vi "Counter (Periodic Tasks).vi"(8 "error in":errorcluster) -> ()   [LabVIEW 2011]
doc: "This VI runs in parallel to other tasks. It can contain as many user-defined periodic loops as you need. These can carry out PID or other sorts of timed response."
uses:
  <vilib>/Rock Robotics/WPI/DriverStation/WPI_DriverStationRobotMode.ctl
  Robot Global Data.vi
  <vilib>/addons/control/pid/pid.llb/PID Control Input Filter (DBL).vi
  <vilib>/addons/control/pid/pid.llb/PID (DBL).vi
  <vilib>/addons/control/pid/NI_PID_pid.lvlib
panel:
  out "Allow Fire":dbl(graph)
  out "Current RPM":dbl(graph)
  in  "Graph Enabled":bool
  out "Counter Value":i32
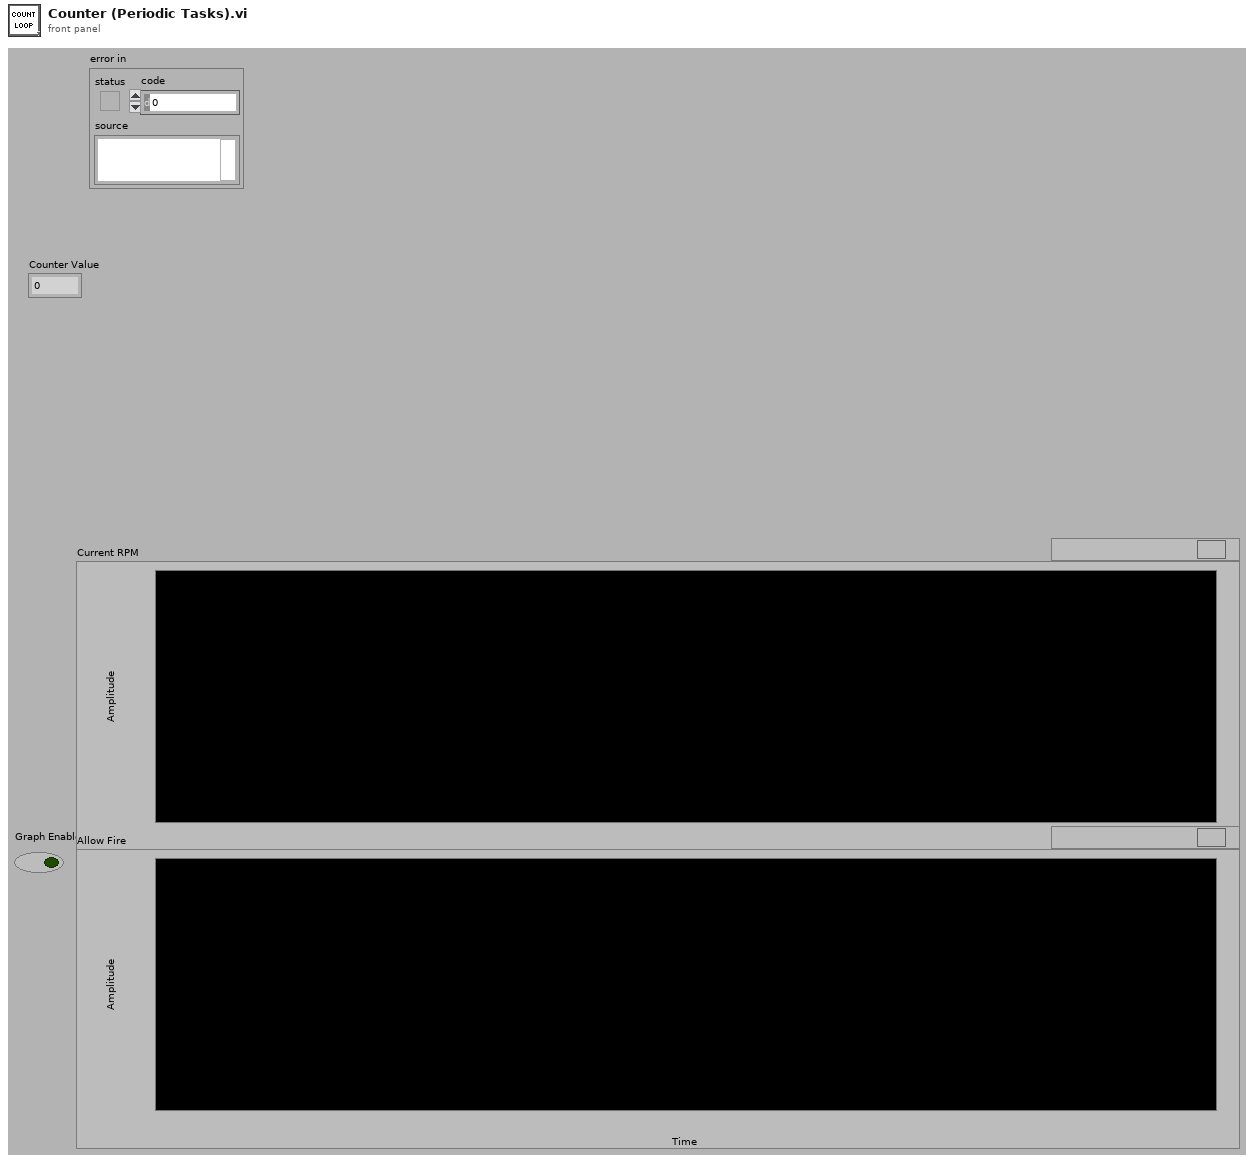
[diagram p1: front panel]
types:
  T1 = typedef "WPI_MotorControlDeviceRef.ctl" = cluster{"DeviceStatus":errorcluster, "Type":enum16{"PWM", "CAN"}, "PWM":cluster{"Digital Module":T2, "PWM Channel":T3, "DeadBand":T4}, "CAN":cluster{"Device Number":u8, "Control Mode":T5, "Semaphore":T6, "Max Vout":dbl}, "Invert":bool, "TransformRef":T7, "InvTransformRef":T7}
  T2 = typedef "FPGA_TypedefDigitalModule.ctl" = enum16{"Digital Module 1", "Digital Module 2"}
  T3 = typedef "FPGA_DIOPWMChannel.ctl" = enum8{"PWM 1", "PWM 2", "PWM 3", "PWM 4", "PWM 5", "PWM 6", "PWM 7", "PWM 8", "PWM 9", "PWM 10", "Invalid"}
  T4 = typedef "WPI_PWMDeadband.ctl" = cluster{"Name":string, "maxPositivePwm":i32, "minPositivePwm":i32, "centerPwm":i32, "maxNegativePwm":i32, "minNegativePwm":i32, "angularRange":u16}
  T5 = typedef "WPI_CANJaguar_ControlMode.ctl" = enum8{"Percent VBus", "Current", "Speed", "Position", "Voltage"}
  T6 = typedef "Semaphore RefNum" = refnum<k1>
  T7 = typedef "WPI_PWMTransform_ConPane.ctl" = refnum<vi>
  T8 = typedef "WPI_CounterDevRef.ctl" = cluster{"DevStatus":errorcluster, "CntIndex":T9}
  T9 = typedef "FPGA_CounterCtrSystemIndex.ctl" = enum8{"Ctr 0", "Ctr 1", "Ctr 2", "Ctr 3", "Ctr 4", "Ctr 5", "Ctr 6", "Ctr 7", "Invalid"}
  T10 = typedef "WPI_DriverStationRobotMode.ctl" = enum16{"Autonomous Disabled", "Autonomous Enabled", "Teleop Disabled", "Teleop Enabled", "Timeout", "Finish"}
  T11 = cluster{"Max Percentage":dbl, "Min Percentage":dbl}
  T12 = cluster{"proportional gain (Kc)":dbl, "integral time (Ti, min)":dbl, "derivative time (Td, min)":dbl}
  T13 = typedef "UDP Dashboard Packet TypeDef.ctl" = cluster{"Distance":dbl, "Shooter Control":cluster{"Manual Enabled":bool, "Manual Distance":dbl, "Power Constant":dbl, "RPM Constant":dbl, "Layup Distance":dbl, "RPM Range":cluster{"Max Percentage":dbl, "Min Percentage":dbl}, "Dt In":dbl}, "Tracking Setpoint":dbl, "Shooter PID gains":cluster{"proportional gain (Kc)":dbl, "integral time (Ti, min)":dbl, "derivative time (Td, min)":dbl}, "Tracking PID gains":cluster{"proportional gain (Kc)":dbl, "integral time (Ti, min)":dbl, "derivative time (Td, min)":dbl}, "Shooter PID gains 2":cluster{"proportional gain (Kc)":dbl, "integral time (Ti, min)":dbl, "derivative time (Td, min)":dbl}, "Tracking Tolerance":dbl, "Tracking Limit":dbl, "Autonomous Ball Collection / Shoot Period":dbl}
  T14 = cluster{"proportional gain (Kc)":dbl, "integral time (Ti, min)":dbl}
  T15 = cluster{"Shooter Warmup":bool, "Shooter Allow Fire":bool}
  T16 = cluster{"Current RPM":dbl, "Distance Setpoint":dbl, "Target RPM":dbl, "Motor Output":dbl, "Base Power":dbl, "Dt Out":dbl}
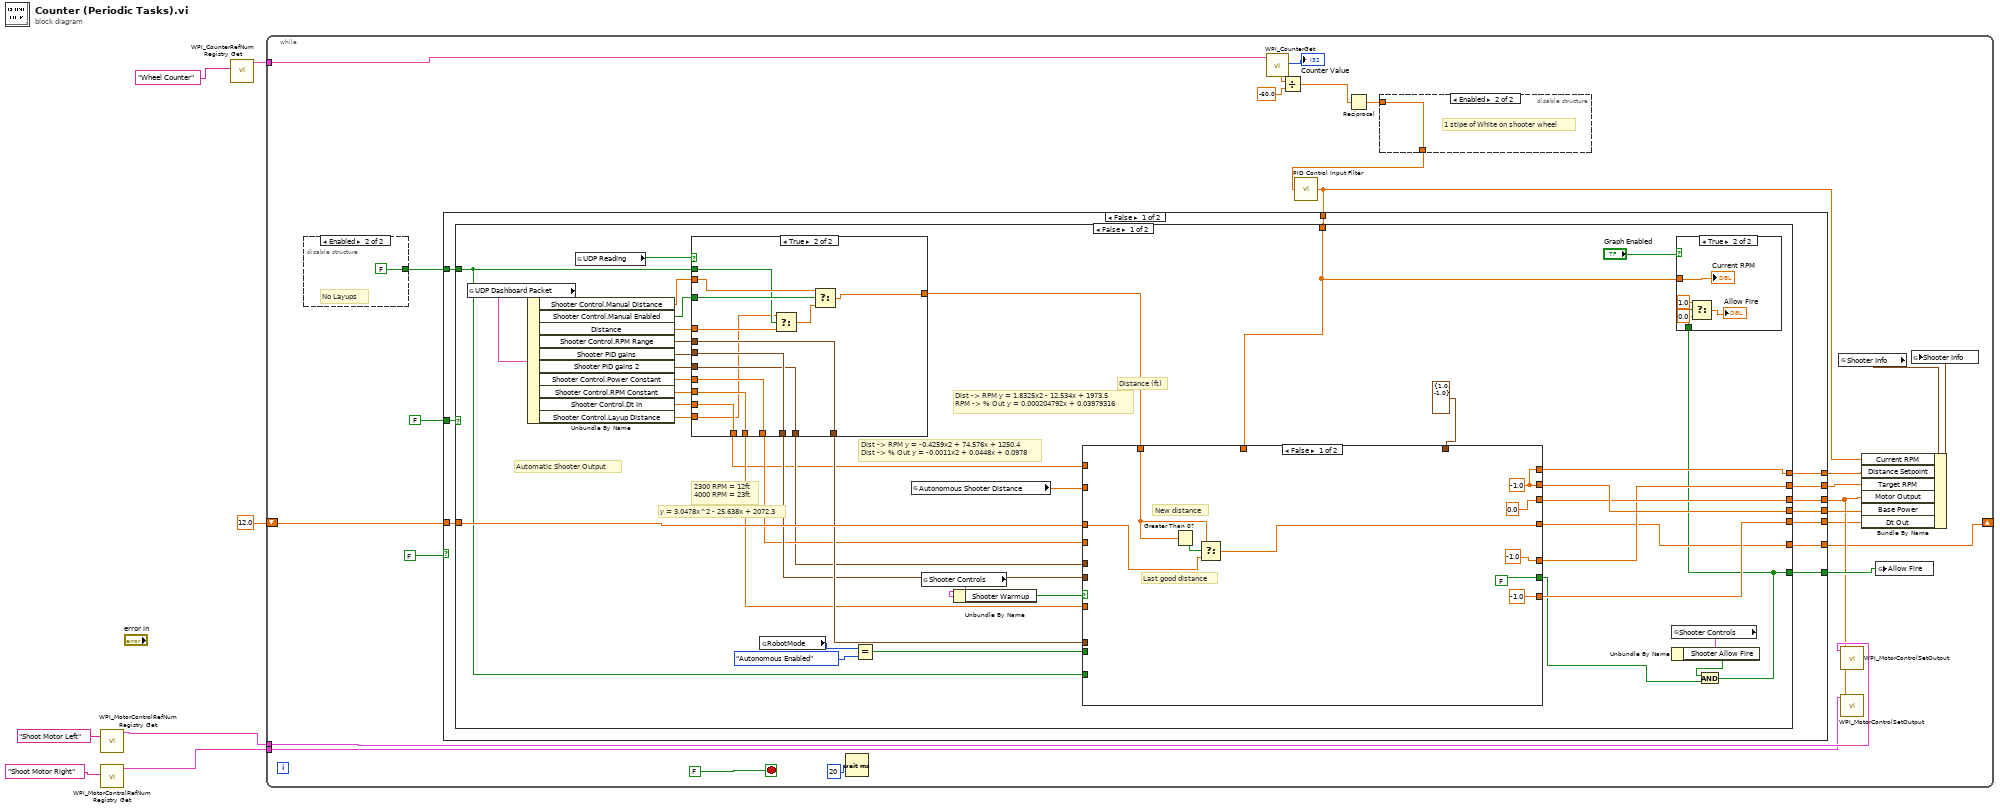
[diagram p0: block diagram]
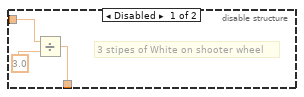
[diagram p2: hidden frame]
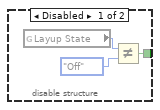
[diagram p3: hidden frame]
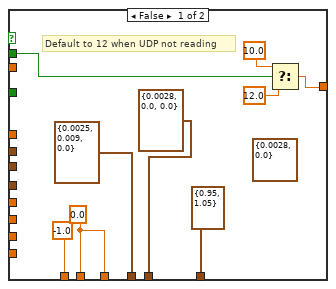
[diagram p4: hidden frame]
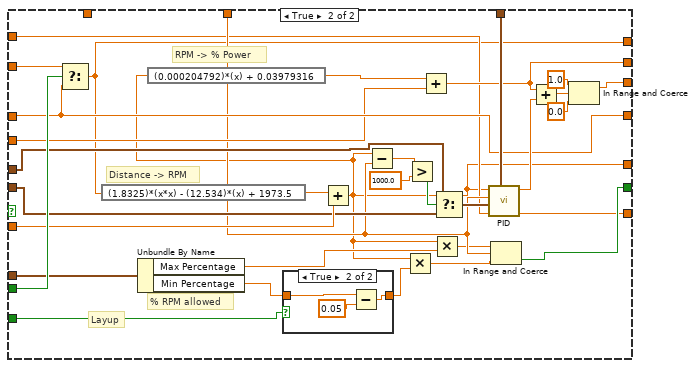
[diagram p6: hidden frame]
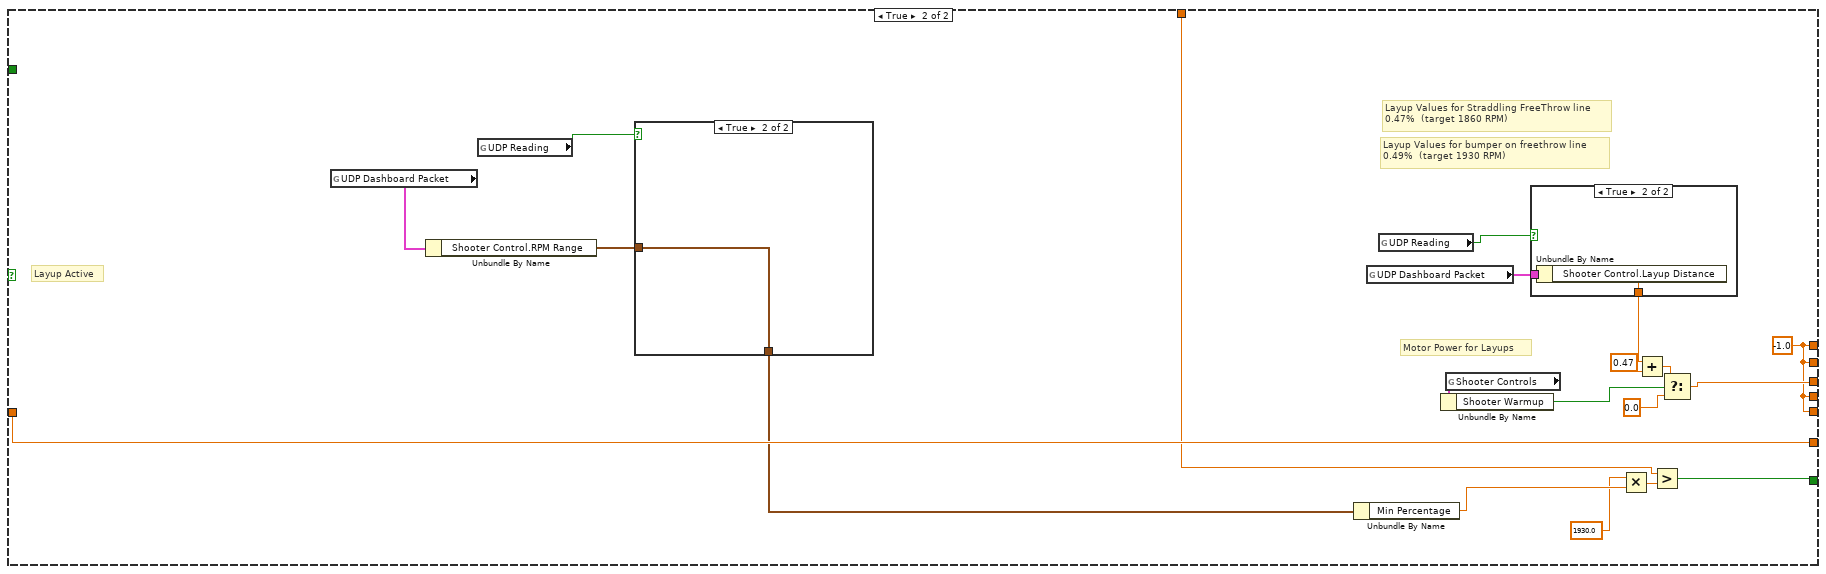
[diagram p8: hidden frame]
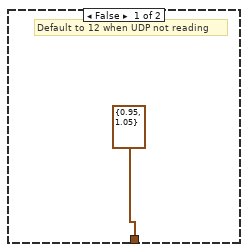
[diagram p9: hidden frame]
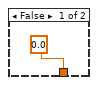
[diagram p10: hidden frame]
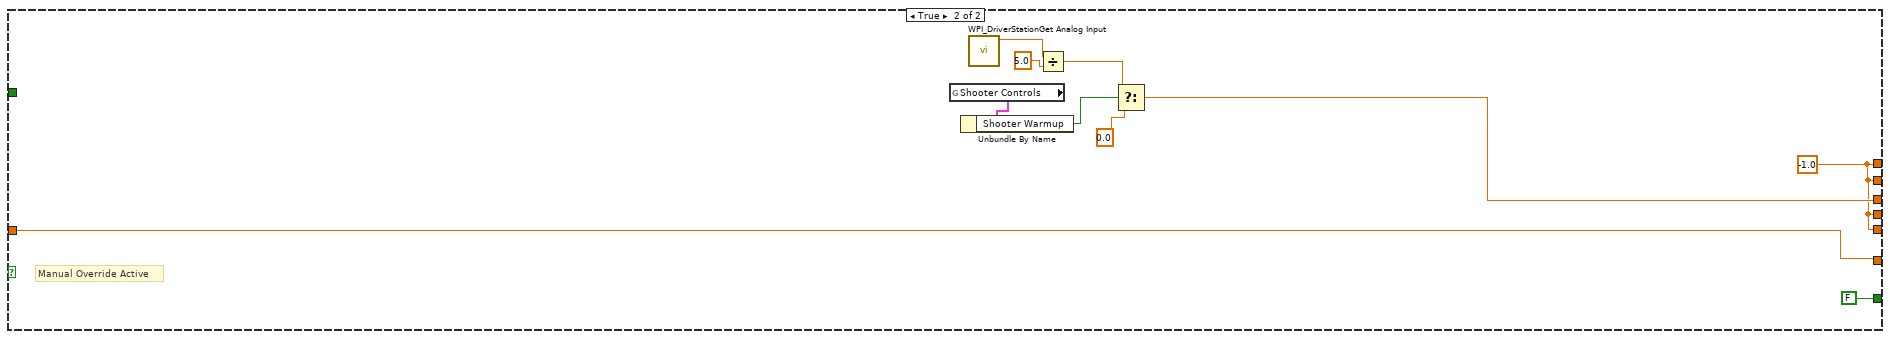
[diagram p11: hidden frame]
diagram:
  n1 = call <vilib>:"WPI_MotorControlRefNum Registry Get.vi"("refnum name"="Shoot Motor Left") -> ("MotorControlDevRef"=w3:T1)  [unwired: 9 in, 1 out]
  n2 = call <vilib>:"WPI_MotorControlRefNum Registry Get.vi"("refnum name"="Shoot Motor Right") -> ("MotorControlDevRef"=w5:T1)  [unwired: 9 in, 1 out]
  n3 = call <vilib>:"WPI_CounterRefNum Registry Get.vi"("refnum name"="Wheel Counter") -> ("CounterDevRef"=w2:T8)  [unwired: 9 in, 1 out]
  n4 = while {
    tunnel: w2 -> [w24]
    tunnel: w3 -> [w30]
    tunnel: w5 -> [w29]
    shift-right: [w14] -> _
    shift-left: 12.0 ("Distance") -> [w28]
    stop <- FALSE stop-if-true
    n5 = disable-structure shown="Enabled" {
      disable-tunnel: [w38 FALSE] -> w15
      frame Disabled {
        n6 = global read "Robot Global Data.vi" "Layup State"() -> (w37:enum16{"Layup Left", "Layup Right", "Off"})
        n7 = Not Equal?(x=w37, y=enum16{"Layup Left", "Layup Right", "Off"}."Off" ("Layup State")) -> (x != y?=w38:bool)
      }
      frame Enabled {
        # "No Layups"
      }
    }
    n8 = Wait (ms)(milliseconds to wait=u32 20) -> ()  [unwired: 1 out]
    n9 = call <vilib>:"WPI_CounterGet.vi"("CounterDevRef in"=w24) -> ("Value"=→"Counter Value":i32, "Period (sec)"=w27:dbl)  [unwired: 5 in, 4 out]
    n10 = Divide(x=w27, y=-60.0) -> (x/y=w10:dbl)
    n11 = Reciprocal(x=w10) -> (1/x=w9:dbl)
    n12 = disable-structure shown="Enabled" {
      disable-tunnel: w9 -> [w34 w36]
      disable-tunnel: [w33 w36] -> w8
      frame Disabled {
        # "3 stipes of White on shooter wheel"
        n13 = Divide(x=w34, y=3.0) -> (x/y=w33:dbl)
      }
      frame Enabled {
        # "1 stipe of White on shooter wheel"
      }
    }
    n14 = call-poly <vilib>:"PID Control Input Filter.vi"("input"=w8) -> ("output"=w17:dbl)  [unwired: 4 in]
    n15 = case shown="False" FALSE ("Boolean") {
      tunnel: w28 -> [w51 w192]
      tunnel: [w47 w192] -> w14
      tunnel: w17 -> [w46 _]
      tunnel: [w50 w193] -> w21
      tunnel: [w49 w195] -> w16
      tunnel: [w48 w193] -> w20
      tunnel: [w44 w193] -> w19
      tunnel: [w45 FALSE] -> w18
      tunnel: w15 -> [w42 _]
      tunnel: [w43 w193] -> w13
      tunnel: FALSE -> [w41 _]
      frame False {
        n16 = case shown="False" w41 {
          tunnel: w51 -> [w91 w184]
          tunnel: [w72 w176] -> w50
          tunnel: [w71 w182] -> w49
          tunnel: [w70 w176] -> w48
          tunnel: [w63 w184] -> w47
          tunnel: w46 -> [w69 w168]
          tunnel: [w56 w167] -> w45
          tunnel: [w58 w176] -> w44
          tunnel: [w64 w176] -> w43
          tunnel: w42 -> [w59 _]
          frame False {
            # "Dist -> RPM y = 1.8325x2 - 12.534x + 1973.5\nRPM -> % Out y = 0.000204792x + 0.03979316"
            # "Automatic Shooter Output"
            # "Dist -> RPM\ty = -0.4259x2 + 74.576x + 1250.4\nDist -> % Out\ty = -0.0011x2 + 0.0448x + 0.0978"
            # "Distance (ft)"
            # "y = 3.0478x^2 - 25.638x + 2072.3"
            # "2300 RPM = 12ft\n4000 RPM = 23ft"
            n17 = global read "Robot Global Data.vi" "UDP Dashboard Packet"() -> (w80:T13)
            n18 = Unbundle By Name(w80) -> ("Shooter Control.Manual Distance"=w76:dbl, "Shooter Control.Manual Enabled"=w84:bool, "Distance"=w85:dbl, "Shooter Control.RPM Range"=w87:T11, "Shooter PID gains"=w88:T12, "Shooter PID gains 2"=w65:T12, "Shooter Control.Power Constant"=w66:dbl, "Shooter Control.RPM Constant"=w67:dbl, "Shooter Control.Dt In"=w61:dbl, "Shooter Control.Layup Distance"=w60:dbl)
            n19 = global read "Robot Global Data.vi" "UDP Reading"() -> (w86:bool)
            n20 = case shown="True" w86 {
              tunnel: w84 -> [_ w109]
              tunnel: w85 -> [_ w104]
              tunnel: [w94 w107] -> w83
              tunnel: w87 -> [_ w113]
              tunnel: [T11 {"Max Percentage"=0.95, "Min Percentage"=1.05} ("RPM Range") w113] -> w82
              tunnel: [T12 {"proportional gain (Kc)"=0.0025, "integral time (Ti, min)"=0.009, "derivative time (Td, min)"=0.0} ("PID gains") w112] -> w81
              tunnel: w88 -> [_ w112]
              tunnel: [w99 w111] -> w78
              tunnel: w66 -> [_ w111]
              tunnel: [w99 w110] -> w77
              tunnel: w67 -> [_ w110]
              tunnel: w76 -> [_ w108]
              tunnel: [T12 {"proportional gain (Kc)"=0.0028, "integral time (Ti, min)"=0.0, "derivative time (Td, min)"=0.0} ("PID gains") w106] -> w68
              tunnel: w65 -> [_ w106]
              tunnel: [-1.0 ("Dt In") w105] -> w62
              tunnel: w61 -> [_ w105]
              tunnel: w59 -> [w95 w102]
              tunnel: w60 -> [_ w101]
              frame False {
                (unwired) T14 {"proportional gain (Kc)"=0.0028, "integral time (Ti, min)"=0.0} ("PID gains")
                w99 = 0.0 ("RPM Constant")
                # "Default to 12 when UDP not reading"
                n21 = Select(t=10.0 ("Manual Distance"), s=w95, f=12.0 ("Manual Distance")) -> (s? t:f=w94:dbl)
              }
              frame True {
                n22 = Select(t=w101, s=w102, f=w104) -> (s? t:f=w103:dbl)
                n23 = Select(t=w108, s=w109, f=w103) -> (s? t:f=w107:dbl)
              }
            }
            n24 = global read "Robot Global Data.vi" "RobotMode"() -> (w75:T10)
            n25 = Equal?(x=w75, y=WPI_DriverStationRobotMode."Autonomous Enabled" ("Robot Mode")) -> (x = y?=w73:bool)
            n26 = global read "Robot Global Data.vi" "Autonomous Shooter Distance"() -> (w79:dbl)
            n27 = global read "Robot Global Data.vi" "Shooter Controls"() -> (w52:T15)
            n28 = Unbundle By Name(w52) -> ("Shooter Warmup"=w55:bool)
            n29 = case shown="False" w55 {
              tunnel: cluster{"output high":dbl, "output low":dbl} {"output high"=1.0, "output low"=-1.0} ("Shooter output range") -> [_ w158]
              tunnel: [0.0 w152] -> w71
              tunnel: [FALSE w135] -> w57
              tunnel: w81 -> [_ w143]
              tunnel: w69 -> [_ w139]
              tunnel: w83 -> [w124 _]
              tunnel: [w122 w153] -> w63
              tunnel: w91 -> [w121 w153]
              tunnel: w82 -> [_ w138]
              tunnel: [-1.0 w128] -> w70
              tunnel: w73 -> [_ w160]
              tunnel: w79 -> [_ w159]
              tunnel: [w119 w151] -> w72
              tunnel: w78 -> [_ w149]
              tunnel: w77 -> [_ w150]
              tunnel: w68 -> [_ w141]
              tunnel: [-1.0 ("dt out (s)") w134] -> w64
              tunnel: w62 -> [_ w133]
              tunnel: w59 -> [_ w130]
              tunnel: [w119 w129] -> w58
              frame False {
                w119 = -1.0
                # "Last good distance"
                # "New distance"
                n30 = Greater Than 0?(x=w124) -> (x > 0?=w123:bool)
                n31 = Select(t=w124, s=w123, f=w121) -> (s? t:f=w122:dbl)
              }
              frame True {
                # "Layup"
                # "Distance -> RPM"
                # "RPM -> % Power"
                # "% RPM allowed"
                n32 = Select(t=w159, s=w160, f=w153) -> (s? t:f=w129:dbl)
                n33 = expression code="(1.8325)*(x*x) - (12.534)*(x) + 1973.5"(w129) -> (w147:dbl)
                n34 = Unbundle By Name(w138) -> ("Max Percentage"=w137:dbl, "Min Percentage"=w132:dbl)
                n35 = case shown="True" w130 {
                  tunnel: w132 -> [w161 w164]
                  tunnel: [w161 w162] -> w131
                  frame False {
                  }
                  frame True {
                    n36 = Subtract(x=w164, y=0.05) -> (x-y=w162:dbl)
                  }
                }
                n37 = Add(x=w147, y=w150) -> (x+y=w128:dbl)
                n38 = expression code="(0.000204792)*(x) + 0.03979316"(w128) -> (w148:dbl)
                n39 = Subtract(x=w128, y=w139) -> (x-y=w146:dbl)
                n40 = Multiply(x=w128, y=w131) -> (x*y=w140:dbl)
                n41 = Greater?(x=w146, y=1000.0) -> (0:w145:bool)
                n42 = Add(x=w148, y=w149) -> (x+y=w151:dbl)
                n43 = Multiply(x=w128, y=w137) -> (x*y=w136:dbl)
                n44 = Select(t=w141, s=w145, f=w143) -> (s? t:f=w142:T12)
                n45 = call-poly <vilib>:"PID.vi"("output range"=w158, "dt (s)"=w133, "PID gains"=w142, "process variable"=w139, "setpoint"=w128) -> ("dt out (s)"=w134:dbl, "output"=w157:dbl)  [unwired: 5 in]
                n46 = In Range and Coerce(upper limit=w136, x=w139, lower limit=w140) -> (In Range?=w135:bool)  [unwired: 1 out]
                n47 = Add(x=w151, y=w157) -> (x+y=w156:dbl)
                n48 = In Range and Coerce(upper limit=1.0, x=w156, lower limit=0.0) -> (coerced(x)=w152:dbl)  [unwired: 1 out]
              }
            }
            n49 = global read "Robot Global Data.vi" "Shooter Controls"() -> (w54:T15)
            n50 = Unbundle By Name(w54) -> ("Shooter Allow Fire"=w53:bool)
            n51 = And(x=w53, y=w57) -> (x .and. y?=w56:bool)
            n52 = case shown="True" "Graph Enabled" {
              tunnel: w69 -> [_ w118]
              tunnel: w56 -> [_ w116]
              frame False {
              }
              frame True {
                n53 = Select(t=1.0, s=w116, f=0.0) -> (s? t:f=→"Allow Fire":dbl)
                "Current RPM" <- w118
              }
            }
          }
          frame True {
            w176 = -1.0 ("Distance")
            # "Layup Values for bumper on freethrow line\n0.49%  (target 1930 RPM)"
            # "Layup Values for Straddling FreeThrow line\n0.47%  (target 1860 RPM)"
            # "Layup Active"
            # "Motor Power for Layups"
            n54 = global read "Robot Global Data.vi" "UDP Dashboard Packet"() -> (w171:T13)
            n55 = Unbundle By Name(w171) -> ("Shooter Control.RPM Range"=w173:T11)
            n56 = global read "Robot Global Data.vi" "UDP Reading"() -> (w172:bool)
            n57 = case shown="True" w172 {
              tunnel: w173 -> [_ w186]
              tunnel: [T11 {"Max Percentage"=0.95, "Min Percentage"=1.05} ("RPM Range") w186] -> w170
              frame False {
                # "Default to 12 when UDP not reading"
              }
              frame True {
              }
            }
            n58 = Unbundle By Name(w170) -> ("Min Percentage"=w175:dbl)
            n59 = global read "Robot Global Data.vi" "UDP Dashboard Packet"() -> (w180:T13)
            n60 = global read "Robot Global Data.vi" "UDP Reading"() -> (w181:bool)
            n61 = global read "Robot Global Data.vi" "Shooter Controls"() -> (w166:T15)
            n62 = Unbundle By Name(w166) -> ("Shooter Warmup"=w165:bool)
            n63 = case shown="True" w181 {
              tunnel: w180 -> [_ w189]
              tunnel: [0.0 ("Layup Power") w188] -> w177
              frame False {
              }
              frame True {
                n64 = Unbundle By Name(w189) -> ("Shooter Control.Layup Distance"=w188:dbl)
              }
            }
            n65 = Multiply(x=1930.0 ("Min Percentage"), y=w175) -> (x*y=w169:dbl)
            n66 = Add(x=w177, y=0.47 ("upper limit")) -> (x+y=w179:dbl)
            n67 = Greater?(x=w168, y=w169) -> (0:w167:bool)
            n68 = Select(t=w179, s=w165, f=0.0) -> (s? t:f=w182:dbl)
          }
        }
      }
      frame True {
        w193 = -1.0 ("Distance Setpoint")
        # "Manual Override Active"
        n69 = global read "Robot Global Data.vi" "Shooter Controls"() -> (w191:T15)
        n70 = Unbundle By Name(w191) -> ("Shooter Warmup"=w190:bool)
        n71 = call <vilib>:"WPI_DriverStationGet Analog Input.vi"() -> ("Analog 1 (V)"=w199:dbl)  [unwired: 8 in, 3 out]
        n72 = Divide(x=w199, y=5.0) -> (x/y=w197:dbl)
        n73 = Select(t=w197, s=w190, f=0.0) -> (s? t:f=w195:dbl)
      }
    }
    n74 = global read "Robot Global Data.vi" "Shooter Info"() -> (w22:T16)
    n75 = call <vilib>:"WPI_MotorControlSetOutput.vi"("Output"=w16, "MotorControlDevRef"=w30) -> ()  [unwired: 8 in, 2 out]
    n76 = call <vilib>:"WPI_MotorControlSetOutput.vi"("Output"=w16, "MotorControlDevRef"=w29) -> ()  [unwired: 8 in, 2 out]
    n77 = Bundle By Name(cluster=w22, "Current RPM"=w17, "Distance Setpoint"=w19, "Target RPM"=w20, "Motor Output"=w16, "Base Power"=w21, "Dt Out"=w13) -> (w23:T16)
    n78 = global write "Robot Global Data.vi" "Allow Fire"(w18) -> ()
    n79 = global write "Robot Global Data.vi" "Shooter Info"(w23) -> ()
  }
